vi "Init_Controls.vi"(8 "Fehler (Eingang, kein Fehler)":errorcluster, 11 "Info Cluster":T2) -> (0 "Fehler (Ausgang)":errorcluster, 3 "first flags out":T1)   [LabVIEW 2020, in "Linearisierung v2.lvlib" / "Gasteiler.lvlib" / "HovaCAL_Interface.lvlib" / "Kommunikation.lvlib"]
uses:
  Kommunikation.lvlib
  Controls/Info Cluster.ctl
  Controls/Controls.lvlib
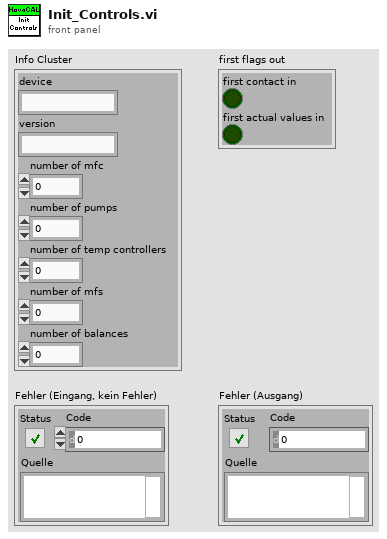
[diagram p1: front panel]
types:
  T1 = cluster{"first contact in":bool, "first actual values in ":bool}
  T2 = typedef "Linearisierung v2.lvlib/Gasteiler.lvlib/HovaCAL_Interface.lvlib/Controls.lvlib/Info Cluster.ctl" = cluster{"device":string, "version":string, "number of mfc":i32, "number of pumps":i32, "number of temp controllers":i32, "number of mfs":i32, "number of balances":i32}
  T3 = cluster{"System Cluster":refnum<vi>, "MFC Flow Cluster":refnum<vi>}
  T4 = cluster{"HovaCAL Limits Cluster":refnum<vi>, "HovaCAL SetPumpMode":refnum<vi>, "HovaCAL Cluster.PumpModeGeneral":refnum<vi>, "HovaCAL SetPumpMode-Cluster":refnum<vi>, "HovaCAL Flow Input Cluster":refnum<vi>, "HovaCAL Set Values Cluster":refnum<vi>[], "HovaCAL Temperature":refnum<vi>, "HovaCAL Pump Concentrations-Cluster":refnum<vi>[], "HovaCAL AutoLin MFC":refnum<vi>, "HovaCAL MFC Gase Cluster Array out":refnum<vi>[]}
  T5 = cluster{"Input Concentration (Ausgang)":refnum<vi>[], "Cluster.Temp Cluster":refnum<vi>, "Cluster.PumpModeGeneral-Cluster":refnum<vi>, "Cluster.Pump Concentrations-Cluster":refnum<vi>[], "Cluster.Flow Output Cluster (Ausgang)":refnum<vi>, "Cluster.Pump MassFlow-Cluster":refnum<vi>, "Cluster.PumpModeGeneral-Cluster 2":refnum<vi>}
  T6 = cluster{"MFC Komponenten Array":refnum<vi>[], "MFC fix + Array":refnum<vi>[]}
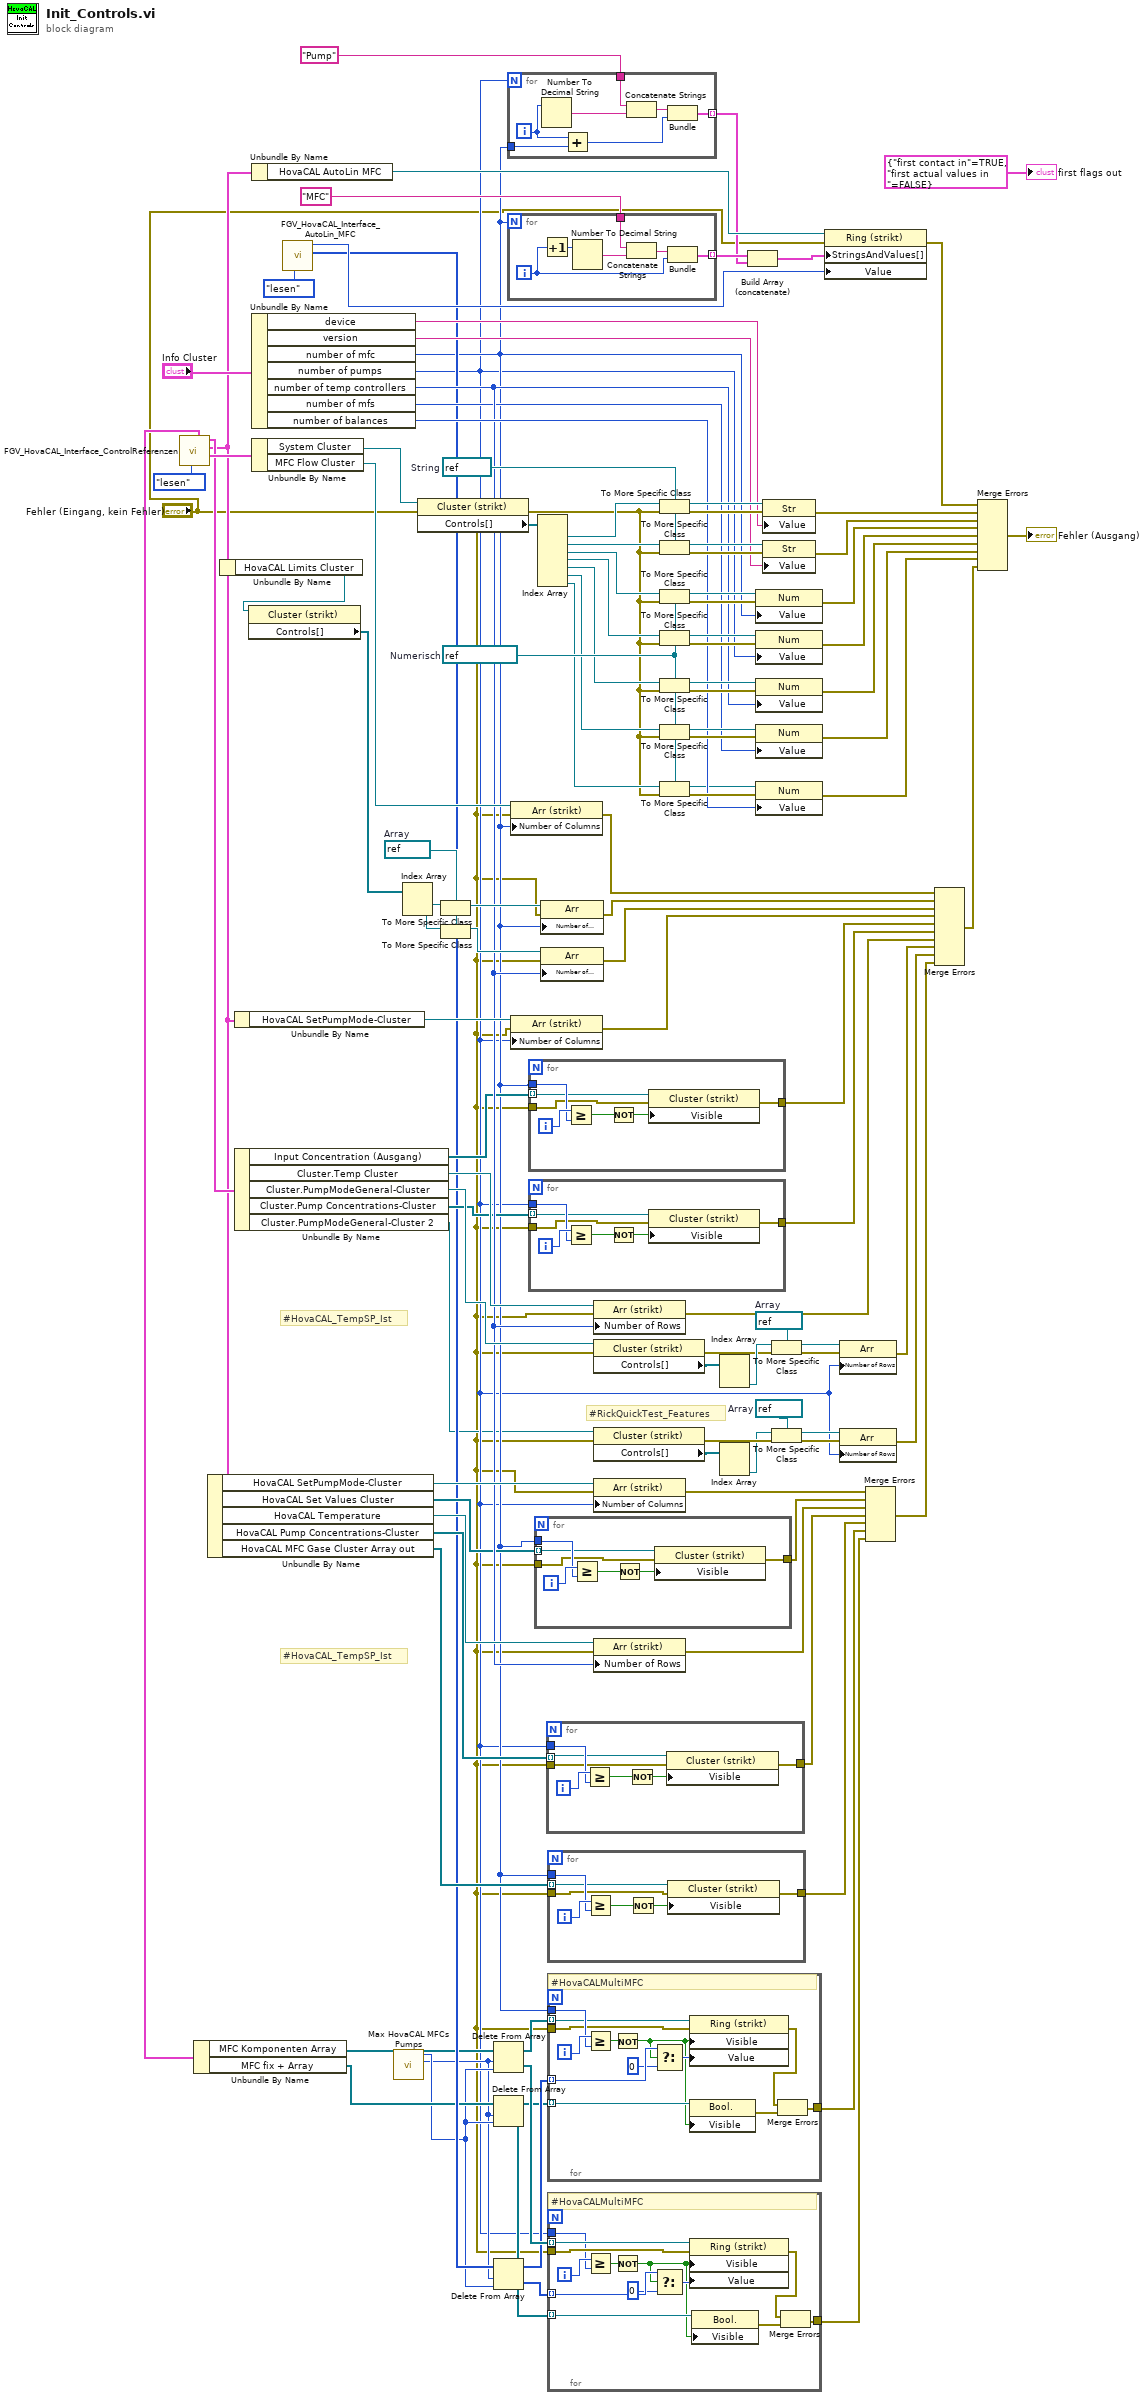
[diagram p0: block diagram]
diagram:
  w6 = refnum<vi> refnum  # Array
  w55 = refnum<vi> refnum  # Array
  w73 = refnum<vi> refnum  # Array
  w93 = refnum<vi> refnum  # Numerisch
  w110 = refnum<vi> refnum  # String
  # "#RickQuickTest_Features"
  # "#HovaCAL_TempSP_Ist"
  # "#HovaCAL_TempSP_Ist"
  n1 = call "FGV_HovaCAL_Interface_ControlReferenzen.vi"("Aktion"=enum16{"lesen", "schreiben"}."lesen") -> ("System Cluster out"=w108:T3, "Set Cluster out"=w49:T4, "Get Cluster out"=w64:T5, "MFC fix Cluster out"=w25:T6)  [unwired: 6 in, 1 out]
  n2 = Unbundle By Name(w25) -> ("MFC Komponenten Array"=w17:refnum<vi>[], "MFC fix + Array"=w16:refnum<vi>[])
  n3 = Unbundle By Name(w49) -> ("HovaCAL SetPumpMode-Cluster"=w48:refnum<vi>, "HovaCAL Set Values Cluster"=w34:refnum<vi>[], "HovaCAL Temperature"=w46:refnum<vi>, "HovaCAL Pump Concentrations-Cluster"=w29:refnum<vi>[], "HovaCAL MFC Gase Cluster Array out"=w36:refnum<vi>[])
  n4 = Unbundle By Name(w49) -> ("HovaCAL Limits Cluster"=w77:refnum<vi>)
  n5 = Unbundle By Name(w49) -> ("HovaCAL SetPumpMode-Cluster"=w67:refnum<vi>)
  n6 = Unbundle By Name(w64) -> ("Input Concentration (Ausgang)"=w31:refnum<vi>[], "Cluster.Temp Cluster"=w59:refnum<vi>, "Cluster.PumpModeGeneral-Cluster"=w57:refnum<vi>, "Cluster.Pump Concentrations-Cluster"=w27:refnum<vi>[], "Cluster.PumpModeGeneral-Cluster 2"=w4:refnum<vi>)
  n7 = property class="Cluster (strikt)"(reference=w77) -> ("Controls[]"=w76:refnum<vi>[])  [unwired: 1 in, 2 out]
  n8 = Unbundle By Name(w49) -> ("HovaCAL AutoLin MFC"=w62:refnum<vi>)
  n9 = Unbundle By Name("Info Cluster") -> ("device"=w106:string, "version"=w105:string, "number of mfc"=w18:i32, "number of pumps"=w5:i32, "number of temp controllers"=w45:i32, "number of mfs"=w40:i32, "number of balances"=w88:i32)
  n10 = Unbundle By Name(w108) -> ("System Cluster"=w107:refnum<vi>, "MFC Flow Cluster"=w78:refnum<vi>)
  n11 = call "FGV_HovaCAL_Interface_AutoLin_MFC.vi"("Aktion"=enum16{"lesen", "schreiben"}."lesen") -> ("MFV Komponente fix out"=w21:u16[], "AutoLin MFC out"=w42:u16)  [unwired: 7 in, 2 out]
  n12 = call "Max HovaCAL MFCs Pumps.vi"() -> ("max Pumps"=w14:i32, "max MFCs"=w15:i32)  [unwired: 10 in]
  n13 = Index Array(array=w76) -> (element #1=w75:refnum<vi>, element #2=w74:refnum<vi>)  [unwired: 2 in]
  n14 = property class="Cluster (strikt)"(reference=w107, error in="Fehler (Eingang, kein Fehler)") -> (error out=w89:errorcluster, "Controls[]"=w116:refnum<vi>[])  [unwired: 1 out]
  n15 = To More Specific Class(target class=w73, reference=w75) -> (specific class reference=w72:refnum<vi>)  [unwired: 1 in, 1 out]
  n16 = To More Specific Class(target class=w73, reference=w74) -> (specific class reference=w71:refnum<vi>)  [unwired: 1 in, 1 out]
  n17 = Delete From Array(array=w17, length=w14, index=w15) -> (deleted portion=w22:refnum<vi>[], array with subset deleted=w24:refnum<vi>[])
  n18 = Delete From Array(array=w16, length=w14, index=w15) -> (deleted portion=w12:refnum<vi>[], array with subset deleted=w13:refnum<vi>[])
  n19 = Delete From Array(array=w21, length=w14, index=w15) -> (deleted portion=w20:u16[], array with subset deleted=w19:u16[])
  n20 = for {
    N: w5 -> [_]
    tunnel: [w125] -> w37 mode=indexing
    tunnel: "Pump" ("String") -> [w121]
    tunnel: w18 -> [w119]
    i -> [w124]
    n21 = Number To Decimal String(number=w124) -> (decimal integer string=w123:string)  [unwired: 1 in]
    n22 = Add(x=w124, y=w119) -> (x+y=w120:i32)
    n23 = Concatenate Strings(w121, w123) -> (w122:string)
    n24 = Bundle(w122, w120) -> (w125:cluster{string, i32})  [unwired: 1 in]
  }
  n25 = for {
    N: w18 -> [_]
    tunnel: [w131] -> w61 mode=indexing
    tunnel: "MFC" ("String") -> [w127]
    i -> [w130]
    n26 = Increment(x=w130) -> (x+1=w126:i32)
    n27 = Number To Decimal String(number=w126) -> (decimal integer string=w129:string)  [unwired: 1 in]
    n28 = Concatenate Strings(w127, w129) -> (w128:string)
    n29 = Bundle(w128, w130) -> (w131:cluster{string, i32})  [unwired: 1 in]
  }
  n30 = property class="Arr (strikt)"(reference=w78, error in="Fehler (Eingang, kein Fehler)", "Number of Columns"=w18) -> (error out=w70:errorcluster)  [unwired: 1 out]
  n31 = property class="Arr (strikt)"(reference=w67, error in="Fehler (Eingang, kein Fehler)", "Number of Columns"=w5) -> (error out=w66:errorcluster)  [unwired: 1 out]
  n32 = for {
    tunnel: w31 -> [w135] mode=indexing
    tunnel: w18 -> [w137]
    tunnel: [w133] -> w32
    tunnel: "Fehler (Eingang, kein Fehler)" -> [w132]
    i -> [w138]
    n33 = Greater Or Equal?(x=w138, y=w137) -> (x >= y?=w136:bool)
    n34 = Not(x=w136) -> (.not. x?=w134:bool)
    n35 = property class="Cluster (strikt)"(reference=w135, error in=w132, "Visible"=w134) -> (error out=w133:errorcluster)  [unwired: 1 out]
  }
  n36 = for {
    tunnel: w27 -> [w142] mode=indexing
    tunnel: w5 -> [w144]
    tunnel: [w140] -> w28
    tunnel: "Fehler (Eingang, kein Fehler)" -> [w139]
    i -> [w145]
    n37 = Greater Or Equal?(x=w145, y=w144) -> (x >= y?=w143:bool)
    n38 = Not(x=w143) -> (.not. x?=w141:bool)
    n39 = property class="Cluster (strikt)"(reference=w142, error in=w139, "Visible"=w141) -> (error out=w140:errorcluster)  [unwired: 1 out]
  }
  n40 = for {
    tunnel: w34 -> [w149] mode=indexing
    tunnel: w18 -> [w151]
    tunnel: [w147] -> w33
    tunnel: "Fehler (Eingang, kein Fehler)" -> [w146]
    i -> [w152]
    n41 = Greater Or Equal?(x=w152, y=w151) -> (x >= y?=w150:bool)
    n42 = Not(x=w150) -> (.not. x?=w148:bool)
    n43 = property class="Cluster (strikt)"(reference=w149, error in=w146, "Visible"=w148) -> (error out=w147:errorcluster)  [unwired: 1 out]
  }
  n44 = Index Array(array=w116) -> (element #1=w114:refnum<vi>, element #2=w112:refnum<vi>, element #3=w103:refnum<vi>, element #4=w94:refnum<vi>, element #5=w92:refnum<vi>, element #6=w91:refnum<vi>, element #7=w90:refnum<vi>)  [unwired: 7 in]
  n45 = property class="Arr"(reference=w72, error in="Fehler (Eingang, kein Fehler)", "Number of Columns"=w18) -> (error out=w69:errorcluster)  [unwired: 1 out]
  n46 = property class="Arr"(reference=w71, error in="Fehler (Eingang, kein Fehler)", "Number of Columns"=w45) -> (error out=w68:errorcluster)  [unwired: 1 out]
  n47 = for {
    tunnel: w5 -> [w158]
    tunnel: [w155] -> w30
    tunnel: "Fehler (Eingang, kein Fehler)" -> [w154]
    tunnel: w29 -> [w153] mode=indexing
    i -> [w159]
    n48 = Greater Or Equal?(x=w159, y=w158) -> (x >= y?=w157:bool)
    n49 = Not(x=w157) -> (.not. x?=w156:bool)
    n50 = property class="Cluster (strikt)"(reference=w153, error in=w154, "Visible"=w156) -> (error out=w155:errorcluster)  [unwired: 1 out]
  }
  n51 = for {
    tunnel: w36 -> [w163] mode=indexing
    tunnel: w18 -> [w165]
    tunnel: "Fehler (Eingang, kein Fehler)" -> [w161]
    tunnel: [w160] -> w35
    i -> [w166]
    n52 = Greater Or Equal?(x=w166, y=w165) -> (x >= y?=w164:bool)
    n53 = Not(x=w164) -> (.not. x?=w162:bool)
    n54 = property class="Cluster (strikt)"(reference=w163, error in=w161, "Visible"=w162) -> (error out=w160:errorcluster)  [unwired: 1 out]
  }
  n55 = for {
    tunnel: w24 -> [w176] mode=indexing
    tunnel: w18 -> [w178]
    tunnel: "Fehler (Eingang, kein Fehler)" -> [w175]
    tunnel: [w168] -> w26
    tunnel: w19 -> [w173] mode=indexing
    tunnel: w13 -> [w170] mode=indexing
    i -> [w179]
    # "#HovaCALMultiMFC"
    n56 = Greater Or Equal?(x=w179, y=w178) -> (x >= y?=w177:bool)
    n57 = Not(x=w177) -> (.not. x?=w169:bool)
    n58 = Select(t=w173, s=w169, f=u16 0) -> (s? t:f=w172:u16)
    n59 = property class="Ring (strikt)"(reference=w176, error in=w175, "Visible"=w169, "Value"=w172) -> (error out=w174:errorcluster)  [unwired: 1 out]
    n60 = property class="Bool."(reference=w170, "Visible"=w169) -> (error out=w167:errorcluster)  [unwired: 1 in, 1 out]
    n61 = Merge Errors(w174, w167) -> (w168:errorcluster)
  }
  n62 = for {
    tunnel: w22 -> [w189] mode=indexing
    tunnel: w5 -> [w188]
    tunnel: "Fehler (Eingang, kein Fehler)" -> [w190]
    tunnel: [w181] -> w23
    tunnel: w20 -> [w187] mode=indexing
    tunnel: w12 -> [w183] mode=indexing
    i -> [w192]
    # "#HovaCALMultiMFC"
    n63 = Greater Or Equal?(x=w192, y=w188) -> (x >= y?=w191:bool)
    n64 = Not(x=w191) -> (.not. x?=w182:bool)
    n65 = Select(t=w187, s=w182, f=u16 0) -> (s? t:f=w186:u16)
    n66 = property class="Ring (strikt)"(reference=w189, error in=w190, "Visible"=w182, "Value"=w186) -> (error out=w180:errorcluster)  [unwired: 1 out]
    n67 = property class="Bool."(reference=w183, "Visible"=w182) -> (error out=w184:errorcluster)  [unwired: 1 in, 1 out]
    n68 = Merge Errors(w180, w184) -> (w181:errorcluster)
  }
  n69 = property class="Arr (strikt)"(reference=w59, error in="Fehler (Eingang, kein Fehler)", "Number of Rows"=w45) -> (error out=w58:errorcluster)  [unwired: 1 out]
  n70 = property class="Cluster (strikt)"(reference=w57, error in="Fehler (Eingang, kein Fehler)") -> (error out=w52:errorcluster, "Controls[]"=w56:refnum<vi>[])  [unwired: 1 out]
  n71 = property class="Cluster (strikt)"(reference=w4, error in="Fehler (Eingang, kein Fehler)") -> (error out=w10:errorcluster, "Controls[]"=w7:refnum<vi>[])  [unwired: 1 out]
  n72 = property class="Arr (strikt)"(reference=w48, error in="Fehler (Eingang, kein Fehler)", "Number of Columns"=w5) -> (error out=w47:errorcluster)  [unwired: 1 out]
  n73 = property class="Arr (strikt)"(reference=w46, error in="Fehler (Eingang, kein Fehler)", "Number of Rows"=w45) -> (error out=w44:errorcluster)  [unwired: 1 out]
  n74 = To More Specific Class(target class=w110, reference=w114, error in=w89) -> (specific class reference=w115:refnum<vi>, error out=w113:errorcluster)
  n75 = To More Specific Class(target class=w110, reference=w112, error in=w89) -> (specific class reference=w111:refnum<vi>, error out=w109:errorcluster)
  n76 = To More Specific Class(target class=w93, reference=w103, error in=w89) -> (specific class reference=w102:refnum<vi>, error out=w104:errorcluster)
  n77 = To More Specific Class(target class=w93, reference=w94, error in=w89) -> (specific class reference=w101:refnum<vi>, error out=w100:errorcluster)
  n78 = To More Specific Class(target class=w93, reference=w92, error in=w89) -> (specific class reference=w98:refnum<vi>, error out=w99:errorcluster)
  n79 = To More Specific Class(target class=w93, reference=w91, error in=w89) -> (specific class reference=w97:refnum<vi>, error out=w96:errorcluster)
  n80 = To More Specific Class(target class=w93, reference=w90, error in=w89) -> (specific class reference=w79:refnum<vi>, error out=w95:errorcluster)
  n81 = Index Array(array=w56) -> (element #2=w54:refnum<vi>)  [unwired: 2 in, 1 out]
  n82 = Index Array(array=w7) -> (element #2=w8:refnum<vi>)  [unwired: 2 in, 1 out]
  n83 = Build Array (concatenate)(w61, w37) -> (w38:cluster{string, i32}[])
  n84 = property class="Num"(reference=w102, error in=w104, "Value"=w18) -> (error out=w84:errorcluster)  [unwired: 1 out]
  n85 = property class="Num"(reference=w101, error in=w100, "Value"=w5) -> (error out=w83:errorcluster)  [unwired: 1 out]
  n86 = property class="Num"(reference=w98, error in=w99, "Value"=w45) -> (error out=w82:errorcluster)  [unwired: 1 out]
  n87 = property class="Num"(reference=w97, error in=w96, "Value"=w40) -> (error out=w81:errorcluster)  [unwired: 1 out]
  n88 = property class="Num"(reference=w79, error in=w95, "Value"=w88) -> (error out=w80:errorcluster)  [unwired: 1 out]
  n89 = property class="Str"(reference=w115, error in=w113, "Value"=w106) -> (error out=w87:errorcluster)  [unwired: 1 out]
  n90 = property class="Str"(reference=w111, error in=w109, "Value"=w105) -> (error out=w85:errorcluster)  [unwired: 1 out]
  n91 = To More Specific Class(target class=w55, reference=w54, error in=w52) -> (specific class reference=w53:refnum<vi>, error out=w51:errorcluster)
  n92 = To More Specific Class(target class=w6, reference=w8, error in=w10) -> (specific class reference=w9:refnum<vi>, error out=w11:errorcluster)
  n93 = property class="Ring (strikt)"(reference=w62, error in="Fehler (Eingang, kein Fehler)", "StringsAndValues[]"=w38, "Value"=w42) -> (error out=w60:errorcluster)  [unwired: 1 out]
  n94 = property class="Arr"(reference=w53, error in=w51, "Number of Rows"=w5) -> (error out=w50:errorcluster)  [unwired: 1 out]
  n95 = property class="Arr"(reference=w9, error in=w11, "Number of Rows"=w5) -> (error out=w1:errorcluster)  [unwired: 1 out]
  n96 = Merge Errors(w47, w33, w44, w30, w35, w26, w23) -> (w2:errorcluster)
  n97 = Merge Errors(w70, w69, w68, w66, w32, w28, w58, w50, w1, w2) -> (w65:errorcluster)
  n98 = Merge Errors(w60, w87, w85, w84, w83, w82, w81, w80, w65) -> (→"Fehler (Ausgang)":errorcluster)
  "first flags out" <- T1 {"first contact in"=TRUE, "first actual values in "=FALSE} ("first flags out")
